vi "Error Handler.vi"(8 "Error in":errorcluster, 10 "From Msg Event":bool, 11 "Core Actor in":refnum<class "Core Actor.lvclass">) -> (0 "Error out":errorcluster, 3 "Core Actor out":refnum<class "Core Actor.lvclass">)   [LabVIEW 2025, in "jettl.lvlib" / "Actor.lvlib" / "Core Actor.lvclass"]
uses:
  Core Actor.lvclass
  Core Actor.lvclass/Core Actor.ctl
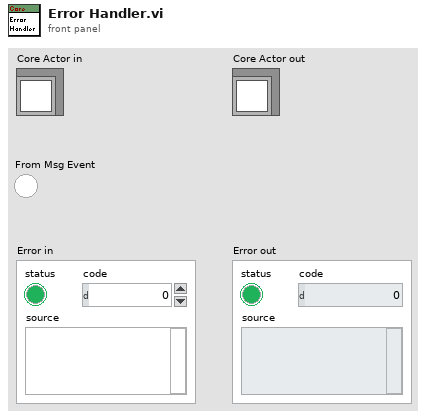
[diagram p1: front panel]
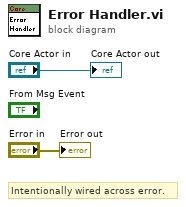
[diagram p0: block diagram]
diagram:
  # "Intentionally wired across error."
  "Core Actor out" <- "Core Actor in"
  "Error out" <- "Error in"
